vi "TCP接收单元.vi"() -> ()   [LabVIEW 2013, in "设备终端.lvclass"]
panel:
  in  "TCP通信功能码":T1(ring)
  in  "设备终端.i":refnum<class "设备终端.lvclass">
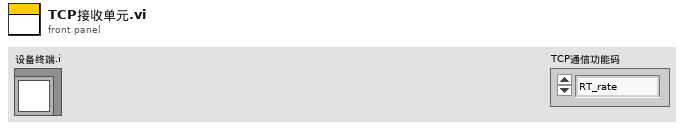
[diagram p1: front panel]
types:
  T1 = enum16{"RT_rate", "RT_dose", "set_th_rate", "set_th_dose", "set_time", "find_div_sign"}
  T2 = enum16{"Standard", "Buffered", "CRLF", "Immediate"}
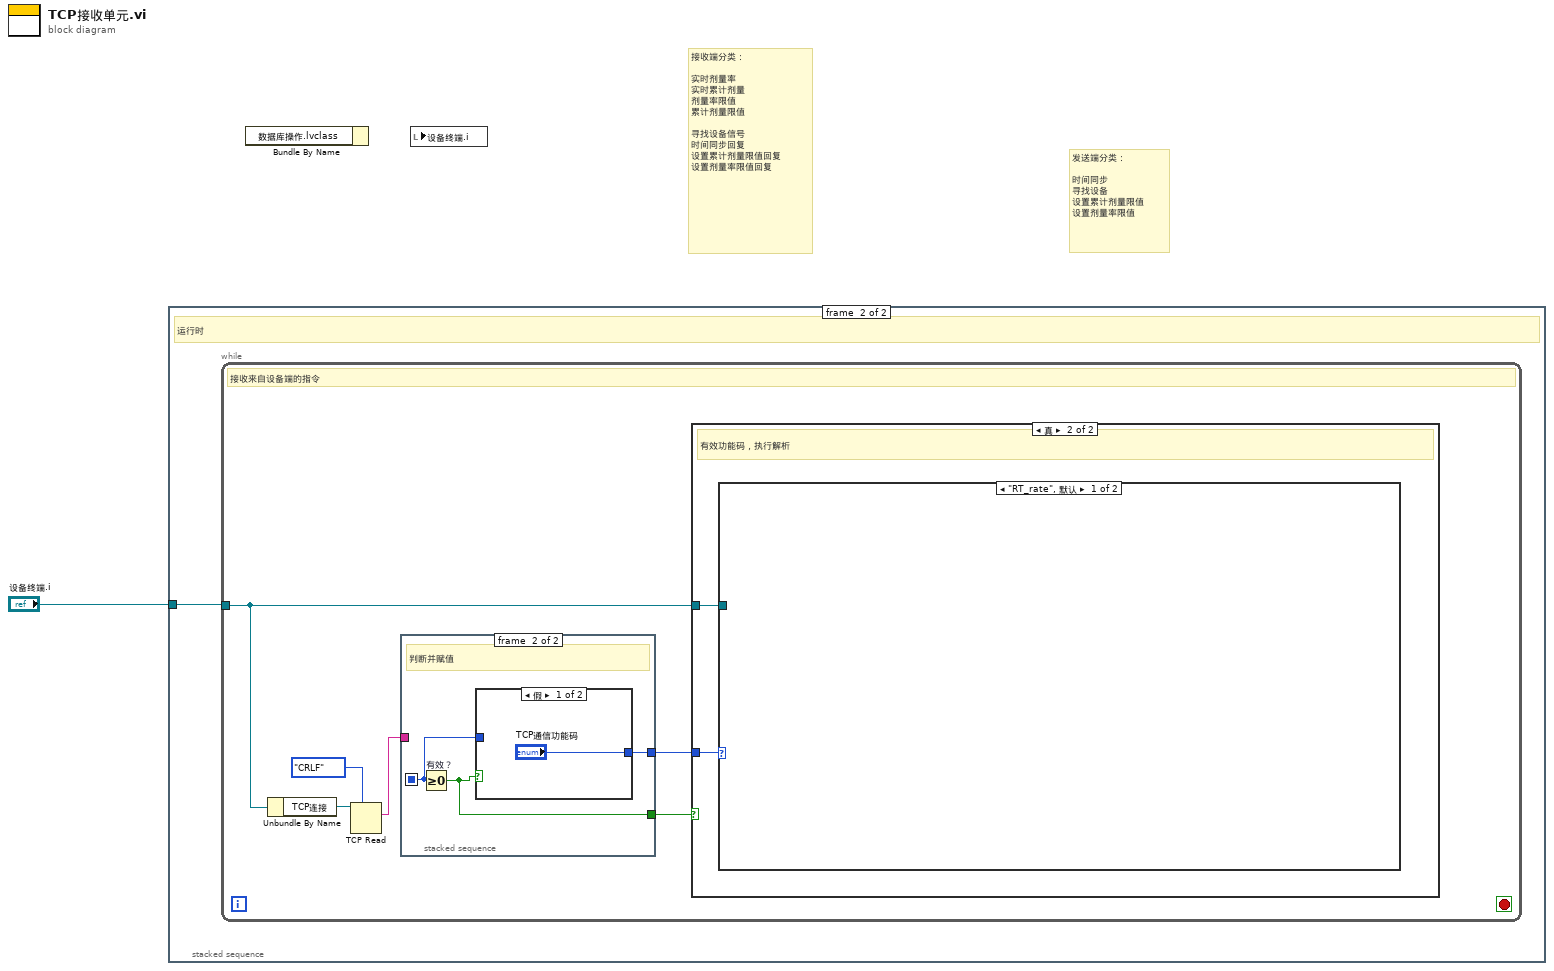
[diagram p0: block diagram]
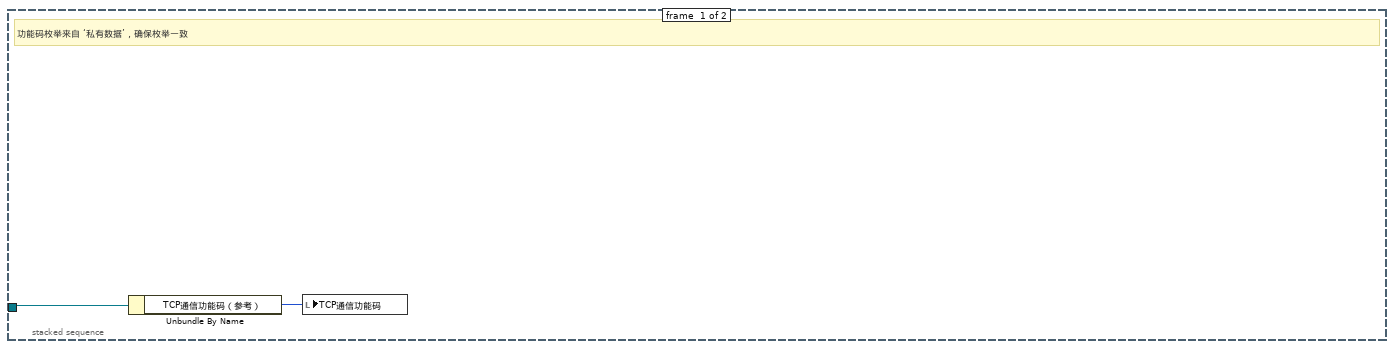
[diagram p2: hidden frame]
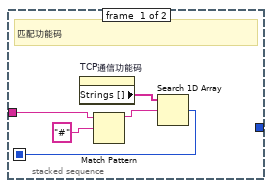
[diagram p5: hidden frame]
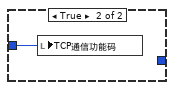
[diagram p6: hidden frame]
diagram:
  # "发送端分类：\n\n时间同步\n寻找设备\n设置累计剂量限值\n设置剂量率限值"
  # "接收端分类：\n\n实时剂量率\n实时累计剂量\n剂量率限值\n累计剂量限值\n\n寻找设备信号\n时间同步回复\n设置累计剂量限值回复\n设置剂量率限值回复"
  n1 = stacked-sequence {
    tunnel: "设备终端.i" -> [w2 w4]
    frame #0 {
      # "功能码枚举来自 ‘私有数据’，确保枚举一致"
      n2 = Unbundle By Name(w2) -> ("TCP通信功能码（参考）"=w3:T1)
      n3 = local write "TCP通信功能码"(w3) -> ()
    }
    frame #1 {
      # "运行时"
      n4 = while {
        tunnel: w4 -> [w8]
        stop <- _ stop-if-true
        # "接收来自设备端的指令"
        n5 = Unbundle By Name(w8) -> ("TCP连接"=w10:refnum<k5>)
        n6 = TCP Read(connection ID=w10, 7:T2."CRLF" ("模式（标准）")) -> (data out=w7:string)  [unwired: 3 in, 2 out]
        n7 = stacked-sequence {
          seq-local: [w13 _] -> [_ w20]
          tunnel: w7 -> [w15 _]
          tunnel: [_ w19] -> w6
          tunnel: [_ w18] -> w5
          frame #0 {
            # "匹配功能码"
            n8 = property on="TCP通信功能码" class="Enum (严格)"() -> ("Strings []"=w17:string[])  [unwired: 2 in, 2 out]
            n9 = Match Pattern(string=w15, regular expression="#" ("正则表达式")) -> (before substring=w14:string)  [unwired: 1 in, 3 out]
            n10 = Search 1D Array(1D array=w17, element=w14) -> (index of element=w13:i32)  [unwired: 1 in]
          }
          frame #1 {
            # "判断并赋值"
            n11 = Greater Or Equal To 0? "有效？"(x=w20) -> (x >= 0?=w18:bool)
            n12 = case shown="假" w18 {
              tunnel: w20 -> [_ w22]
              tunnel: ["TCP通信功能码" _] -> w19
              frame False {
              }
              frame True {
                n13 = local write "TCP通信功能码"(w22) -> ()
              }
            }
          }
        }
        n14 = case shown="真" w5 {
          tunnel: w8 -> [_ w12]
          tunnel: w6 -> [_ w11]
          frame False {
            # "无效功能码，不执行"
          }
          frame True {
            # "有效功能码，执行解析"
            n15 = case shown="\"RT_rate\", 默认" w11 {
              tunnel: w12 -> [_ _]
              frame "RT_rate", Default {
              }
              frame "RT_dose" {
              }
            }
          }
        }
      }
    }
  }
  n16 = Bundle By Name() -> ()  [unwired: 2 in, 1 out]
  n17 = local read "设备终端.i"() -> ()  [unwired: 1 in]
